vi "Read Polarity.vi"(6 "error in":errorcluster, 8 "MaxRead":i32, 9 "Channel in":u16) -> (0 "error out":errorcluster, 1 "Messages":T1(array[cluster]), 2 "Pass":bool, 3 "Channel out":u16)   [LabVIEW 2023]
uses:
  Communication/PCAN2023/PCAN API.lvlib
  e0e8a07b-84dc-4093-b6df-003bb8198d0c.vi
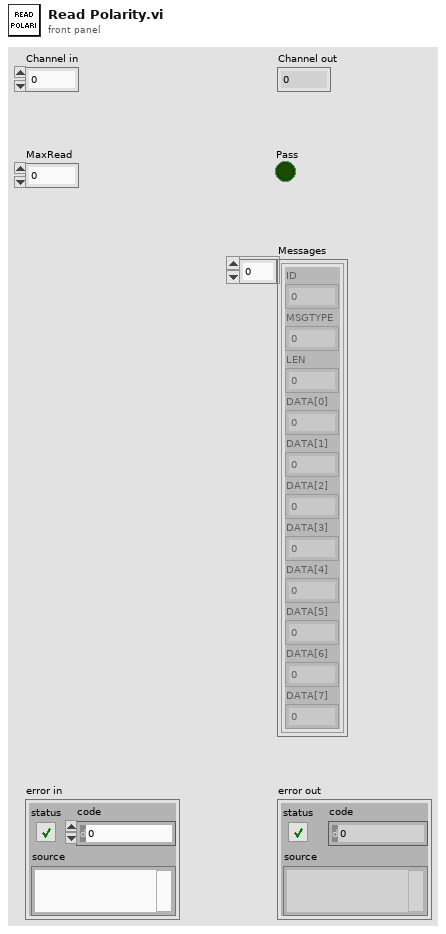
[diagram p1: front panel]
types:
  T1 = cluster{"ID":u32, "MSGTYPE":u8, "LEN":u8, "DATA[0]":u8, "DATA[1]":u8, "DATA[2]":u8, "DATA[3]":u8, "DATA[4]":u8, "DATA[5]":u8, "DATA[6]":u8, "DATA[7]":u8}[]
  T2 = cluster{"ID":u32, "MSGTYPE":u8, "LEN":u8, "DATA[0]":u8, "DATA[1]":u8, "DATA[2]":u8, "DATA[3]":u8, "DATA[4]":u8, "DATA[5]":u8, "DATA[6]":u8, "DATA[7]":u8}
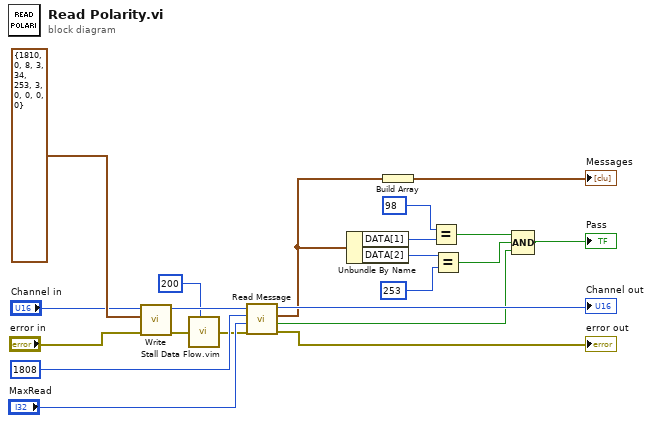
[diagram p0: block diagram]
diagram:
  n1 = call "Write.vi"("error in"="error in", "MessageBuffer"=T2 {"ID"=1810, "MSGTYPE"=0, "LEN"=8, "DATA[0]"=3, "DATA[1]"=34, "DATA[2]"=253, "DATA[3]"=3, "DATA[4]"=0, "DATA[5]"=0, "DATA[6]"=0, "DATA[7]"=0}, "Channel"="Channel in") -> ("error out"=w7:errorcluster, "Channel out"=w10:u16)  [unwired: 5 in, 2 out]
  n2 = call "Stall Data Flow.vim"("value in"=w7, "milliseconds to wait"=u32 200) -> ("value out"=w2:errorcluster)  [unwired: 1 out]
  n3 = call "Read Message.vi"("error in"=w2, "MaxRead"="MaxRead", "ID"=u32 1808, "Channel in"=w10) -> ("error out"=→"error out":errorcluster, "Passed"=w4:bool, "Last Message"=w3:T2, "Channel out"=→"Channel out":u16)  [unwired: 3 in, 1 out]
  n4 = Unbundle By Name(w3) -> ("DATA[1]"=w18:u8, "DATA[2]"=w16:u8)
  n5 = Build Array(w3) -> (→"Messages":T1)
  n6 = Equal?(x=u8 98, y=w18) -> (x = y?=w14:bool)
  n7 = Equal?(x=w16, y=u8 253 ("x")) -> (x = y?=w13:bool)
  n8 = Compound Arithmetic op=AND(w14, w13, w4) -> (→"Pass":bool)
